vi "tcp_query.vi"() -> ()   [LabVIEW 2019]
panel:
  out "client_step":i32
  out "raw string":string
  out "error out":errorcluster
  in  "stop_query":bool
  out "spill_id":i32
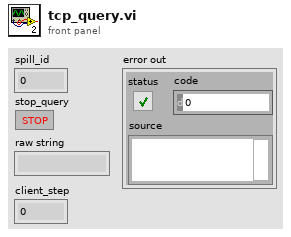
[diagram p1: front panel]
types:
  T1 = enum16{"Standard", "Buffered", "CRLF", "Immediate"}
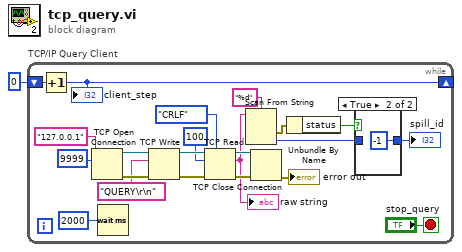
[diagram p0: block diagram]
diagram:
  n1 = while "TCP/IP Query Client" {
    shift-right: [w5] -> _
    shift-left: 0 -> [w6]
    stop <- "stop_query" stop-if-true
    n2 = Increment(x=w6) -> (x+1=w5:i32)
    "client_step" <- w5
    n3 = TCP Open Connection(address="127.0.0.1", remote port or service name=u16 9999) -> (connection ID=w20:refnum<k5>, error out=w19:errorcluster)  [unwired: 3 in]
    n4 = Wait (ms)(milliseconds to wait=u32 2000) -> ()  [unwired: 1 out]
    n5 = TCP Write(connection ID=w20, data in="QUERY\r\n", error in (no error)=w19) -> (connection ID out=w16:refnum<k5>, error out=w17:errorcluster)  [unwired: 1 in, 1 out]
    n6 = TCP Read(connection ID=w16, bytes to read=100, error in (no error)=w17, 7:T1."CRLF" ("mode (standard)")) -> (connection ID out=w14:refnum<k5>, data out=w12:string, error out=w15:errorcluster)  [unwired: 1 in]
    "raw string" <- w12
    n7 = Scan From String(format string="%d", input string=w12) -> (error out=w10:errorcluster, output 1=w7:i32)  [unwired: 3 in, 2 out]
    n8 = TCP Close Connection(connection ID=w14, error in (no error)=w15) -> (error out=→"error out":errorcluster)  [unwired: 1 in, 1 out]
    n9 = Unbundle By Name(w10) -> ("status"=w9:bool)
    n10 = case shown="True" w9 {
      tunnel: [w24 -1] -> w8
      tunnel: w7 -> [w24 _]
      frame False {
      }
      frame True {
      }
    }
    "spill_id" <- w8
  }
